vi "Stable.vi"(8 "Eval Period (sec)":dbl(knob)=0.5044674819294696 scale=0.0..1.0, 11 "Signal Input":bool) -> (0 "Stable":bool)   [LabVIEW 2016]
doc: "Help by FRC Team 836 - The RoboBees\n\nThis will check if a Boolean stays 'on' for a settable pulse width, and outputs a 'Stable' Boolean when this condition is met.\nThe output STABLE is false while the input SIGNAL INPUT is false, and remains false until SIGNAL INPUT has been true\nfor the entire time period designated by EVAL PERIOD (beginning with the rising-edge of SIGNAL INPUT). Once STABLE \nturns true, it remains true for as long as SIGNAL INPUT remains true.\n\nAny SIGNAL INPUT return to false event returns a false STABLE output and resets the evaluation period.\n\nUseful to determine if a boolean condition has stabilized before taking subsequent action."
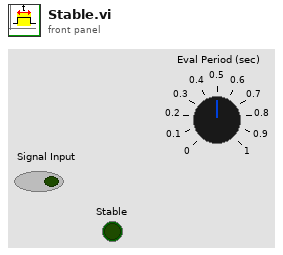
[diagram p1: front panel]
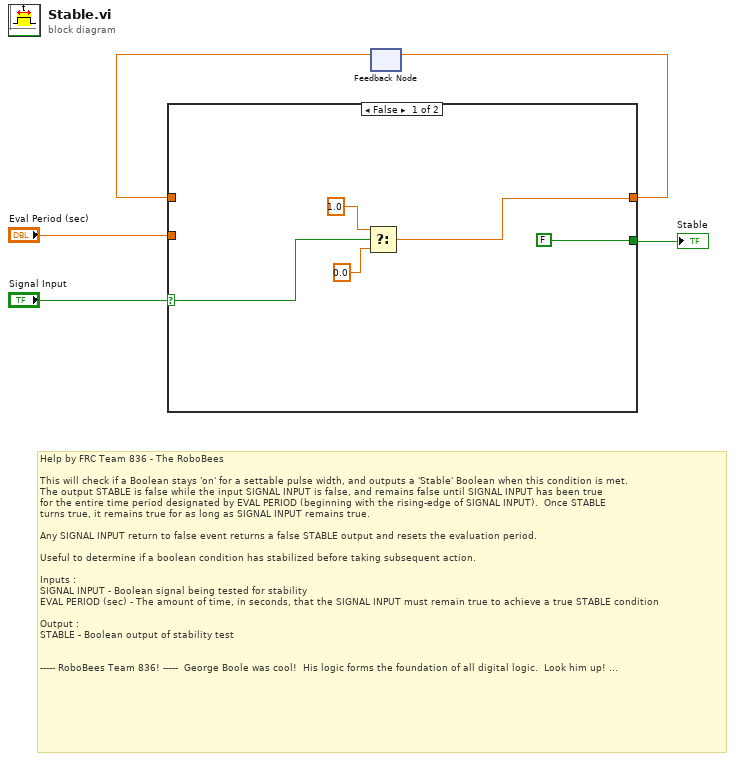
[diagram p0: block diagram]
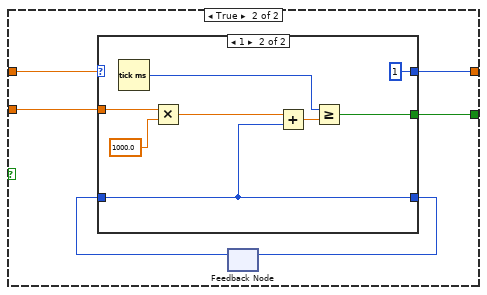
[diagram p2: hidden frame]
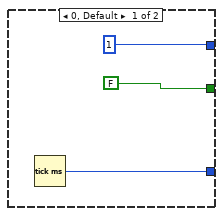
[diagram p3: hidden frame]
diagram:
  # "Help by FRC Team 836 - The RoboBees\n\nThis will check if a Boolean stays 'on' for a settable pulse width, and outputs a 'Stable' Boolean when this condition is met.\nThe output STABLE is false while the input SIGNAL INPUT is false, and remains false until SIGNAL INPUT has been true\nfor the entire time period designated by EVAL PERIOD (beginning with the rising-edge of SIGNAL INPUT).  Once STABLE \nturns true, it remains true for as long as SIGNAL INPUT remains true.\n\nAny SIGNAL INPUT return to false event returns a false STABLE output and resets the evaluation period.\n\nUseful to determine if a boolean condition has stabilized before taking subsequent action.\n\nInputs :\nSIGNAL INPUT - Boolean signal being tested for stability\nEVAL PERIOD (sec) - The amount of time, in seconds, that the SIGNAL INPUT must remain true to achieve a true STABLE condition\n\nOutput :\nSTABLE - Boolean output of stability test\n\n\n----- RoboBees Team 836! -----  George Boole was cool!  His logic forms the foundation of all digital logic.  Look him up! ..."
  n1 = feedback #1() -> (w1:dbl)  [unwired: 1 in]
  n2 = case shown="False" "Signal Input" {
    selector: "Signal Input" -> [w9 _]
    tunnel: [FALSE w16] -> w5
    tunnel: "Eval Period (sec)" -> [_ w15]
    tunnel: [w6 w12] -> w2
    tunnel: w1 -> [_ w11]
    frame False {
      n3 = Select(t=1.0, s=w9, f=0.0) -> (s? t:f=w6:dbl)
    }
    frame True {
      n4 = feedback #2() -> (w13:u32)  [unwired: 1 in]
      n5 = case shown="1" w11 {
        tunnel: [FALSE w26] -> w16
        tunnel: w15 -> [_ w22]
        tunnel: [w17 w25] -> w14
        tunnel: w13 -> [_ w25]
        tunnel: [1 1] -> w12
        frame 0, Default {
          n6 = Tick Count (ms)() -> (millisecond timer value=w17:u32)
        }
        frame 1 {
          n7 = Tick Count (ms)() -> (millisecond timer value=w20:u32)
          n8 = Multiply(x=w22, y=1000.0) -> (x*y=w23:dbl)
          n9 = Add(x=w23, y=w25) -> (x+y=w27:dbl)
          n10 = Greater Or Equal?(x=w20, y=w27) -> (x >= y?=w26:bool)
        }
      }
      n11 = feedback-in #2(w14) -> ()
    }
  }
  "Stable" <- w5
  n12 = feedback-in #1(w2) -> ()
